vi "WPI_RelayClose.vi"(8 "error in (no error)":errorcluster, 11 "RelayDevRef":T1={"DevStatus"={"status"=FALSE, "code"=0, "source"=""}, "Relay Channel"=enum."Invalid", "Relay Direction"=enum."Both directions"}) -> (0 "error out":errorcluster)   [LabVIEW 2017]
doc: "Closes the reference to the relay you specify. Use this VI to close each relay reference that you open with the Open VI.\n\nThis software is licensed. Open the labview\\readme\\WPI Robotics Library Open Source License.txt file for more information."
uses:
  <vilib>/Rock Robotics/WPI/Relay/WPI_RelayDevRef.ctl
  <vilib>/Rock Robotics/SystemInterfaces/DIO/FPGA_DIORelayChannel.ctl
  <vilib>/Rock Robotics/WPI/Relay/WPI_RelayDirection.ctl
  <vilib>/Rock Robotics/WPI/Relay/WPI_RelayCacheOp.ctl
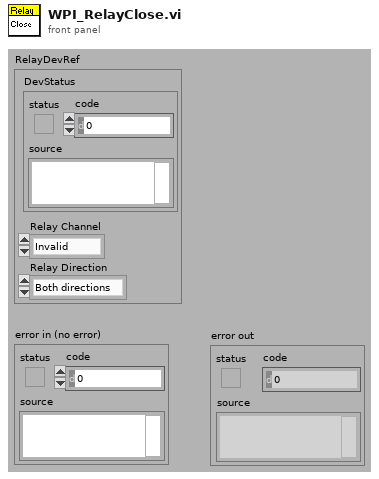
[diagram p1: front panel]
types:
  T1 = typedef "WPI_RelayDevRef.ctl" = cluster{"DevStatus":errorcluster, "Relay Channel":T2, "Relay Direction":T3}
  T2 = typedef "FPGA_DIORelayChannel.ctl" = enum8{"Relay 0", "Relay 1", "Relay 2", "Relay 3", "Invalid"}
  T3 = typedef "WPI_RelayDirection.ctl" = enum16{"Both directions", "Forward only", "Reverse only"}
  T4 = typedef "WPI_RelayCacheOp.ctl" = enum16{"Acquire", "Release", "Status"}
  T5 = typedef "WPI_DigitalModuleDeviceRef.ctl" = cluster{"DevStatus":errorcluster}
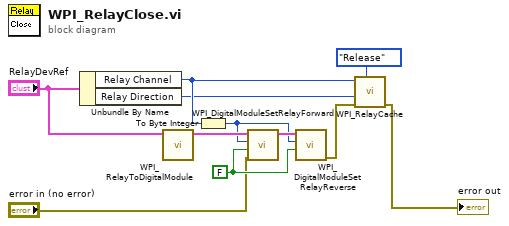
[diagram p0: block diagram]
diagram:
  w10 = FALSE ("Set")
  n1 = Unbundle By Name("RelayDevRef") -> ("Relay Channel"=w7:T2, "Relay Direction"=w3:T3)
  n2 = call <vilib>:"WPI_RelayToDigitalModule.vi"("RelayDevRef"="RelayDevRef") -> ("DigitalModuleDevRef"=w9:T5)  [unwired: 10 out]
  n3 = To Byte Integer(number=w7) -> (8bit integer=w6:i8)
  n4 = call <vilib>:"WPI_DigitalModuleSetRelayForward.vi"("error in (no error)"="error in (no error)", "Value"=w10, "RelayChannel"=w6, "DigitalModuleDevRef"=w9) -> ("DigitalModuleDevRef"=w8:T5)  [unwired: 7 out]
  n5 = call <vilib>:"WPI_DigitalModuleSetRelayReverse.vi"("Value"=w10, "RelayChannel"=w6, "DigitalModuleDevRef"=w8) -> ("error out"=w5:errorcluster)  [unwired: 1 in, 7 out]
  n6 = call <vilib>:"WPI_RelayCache.vi"("Operation"=WPI_RelayCacheOp."Release", "error in (no error)"=w5, "RelayDirection"=w3, "RelayChannelIn"=w7) -> ("error out"=→"error out":errorcluster)  [unwired: 1 in, 6 out]
